vi "TurnXDegrees.vi"(8 "error in (no error)":errorcluster, 9 "Reset?":bool, 10 "degrees":dbl, 11 "RobotDriveDevRef":T1={"DevStatus"={"status"=FALSE, "code"=0, "source"=""}, "Motors[]"=[], "Square Inputs"=FALSE, "Max Output"=1.0, "Isochronous"=FALSE}) -> (0 "error out":errorcluster, 2 "Running":bool)   [LabVIEW 2013]
uses:
  <vilib>/Rock Robotics/WPI/RobotDrive/WPI_RobotDriveDevRef.ctl
  <vilib>/Rock Robotics/WPI/MotorControl/WPI_MotorControlDeviceRef.ctl
  <vilib>/Rock Robotics/SystemInterfaces/Typedef/FPGA_TypedefDigitalModule.ctl
  <vilib>/Rock Robotics/SystemInterfaces/DIO/FPGA_DIOPWMChannel.ctl
  <vilib>/Rock Robotics/WPI/PWM/WPI_PWMDeadband.ctl
  <vilib>/Rock Robotics/WPI/CAN/Jaguar/SubVIs/WPI_CANJaguar_ControlMode.ctl
  <vilib>/Rock Robotics/WPI/PWM/WPI_PWMTransform_ConPane.ctl
  <vilib>/addons/control/pid/pid.llb/PID Control Input Filter (DBL).vi
  <vilib>/addons/control/pid/pid.llb/PID (DBL).vi
  <vilib>/Rock Robotics/WPI/RobotDrive/WPI_RobotDriveArcadeDrive_Standard(NoSaturation).vi
  <vilib>/addons/control/pid/NI_PID_pid.lvlib
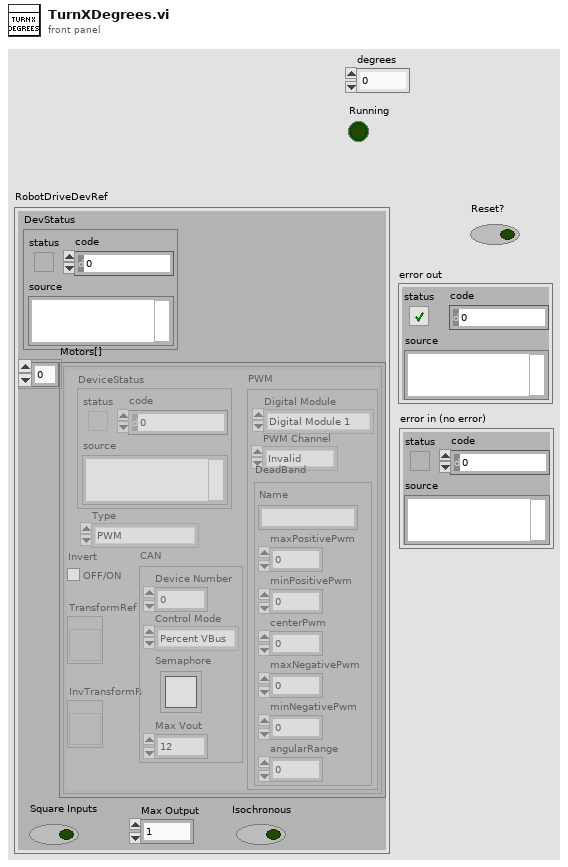
[diagram p1: front panel]
types:
  T1 = typedef "WPI_RobotDriveDevRef.ctl" = cluster{"DevStatus":errorcluster, "Motors[]":T2[], "Square Inputs":bool, "Max Output":dbl, "Isochronous":bool}
  T2 = typedef "WPI_MotorControlDeviceRef.ctl" = cluster{"DeviceStatus":errorcluster, "Type":enum16{"PWM", "CAN"}, "PWM":cluster{"Digital Module":T3, "PWM Channel":T4, "DeadBand":T5}, "CAN":cluster{"Device Number":u8, "Control Mode":T6, "Semaphore":T7, "Max Vout":dbl}, "Invert":bool, "TransformRef":T8, "InvTransformRef":T8}
  T3 = typedef "FPGA_TypedefDigitalModule.ctl" = enum16{"Digital Module 1", "Digital Module 2"}
  T4 = typedef "FPGA_DIOPWMChannel.ctl" = enum8{"PWM 1", "PWM 2", "PWM 3", "PWM 4", "PWM 5", "PWM 6", "PWM 7", "PWM 8", "PWM 9", "PWM 10", "Invalid"}
  T5 = typedef "WPI_PWMDeadband.ctl" = cluster{"Name":string, "maxPositivePwm":i32, "minPositivePwm":i32, "centerPwm":i32, "maxNegativePwm":i32, "minNegativePwm":i32, "angularRange":u16}
  T6 = typedef "WPI_CANJaguar_ControlMode.ctl" = enum8{"Percent VBus", "Current", "Speed", "Position", "Voltage"}
  T7 = typedef "Semaphore RefNum" = refnum<k1>
  T8 = typedef "WPI_PWMTransform_ConPane.ctl" = refnum<vi>
  T9 = cluster{"proportional gain (Kc)":dbl, "integral time (Ti, min)":dbl, "derivative time (Td, min)":dbl}
  T10 = typedef "WPI_GyroDevRef.ctl" = cluster{"DevStatus":errorcluster, "Analog Module":T11, "Analog Channel":T12, "Offset":dbl, "Gain (VoltsPerDegree/Second)":dbl}
  T11 = typedef "FPGA_TypedefAnalogModule.ctl" = enum16{"Analog Module 1", "Analog Module 2"}
  T12 = typedef "FPGA_AIChannel.ctl" = enum8{"AI 1", "AI 2", "AI 3", "AI 4", "AI 5", "AI 6", "AI 7", "AI 8", "Invalid"}
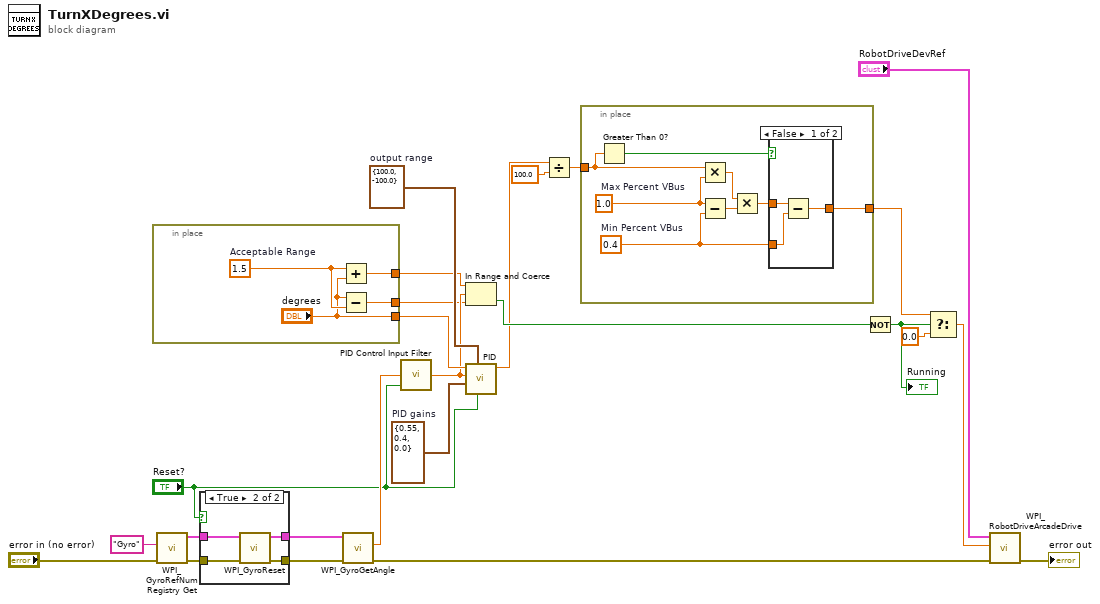
[diagram p0: block diagram]
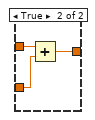
[diagram p2: hidden frame]
diagram:
  w15 = T9 {"proportional gain (Kc)"=0.55, "integral time (Ti, min)"=0.4, "derivative time (Td, min)"=0.0}  # PID gains
  w16 = cluster{"output high":dbl, "output low":dbl} {"output high"=100.0, "output low"=-100.0}  # output range
  n1 = in-place {
    in-place-border: [w28] -> w10
    in-place-border: [w27] -> w9
    in-place-border: ["degrees"] -> w12
    w29 = 1.5  # Acceptable Range
    n2 = Add(x=w29, y="degrees") -> (x+y=w28:dbl)
    n3 = Subtract(x="degrees", y=w29) -> (x-y=w27:dbl)
  }
  n4 = call <vilib>:"WPI_GyroRefNum Registry Get.vi"("error in (no error)"="error in (no error)", "refnum name"="Gyro") -> ("error out"=w21:errorcluster, "GyroDevRef"=w22:T10)  [unwired: 8 in]
  n5 = case shown="True" "Reset?" {
    tunnel: w22 -> [w31 w34]
    tunnel: w21 -> [w30 w35]
    tunnel: [w31 w33] -> w19
    tunnel: [w30 w32] -> w20
    frame False {
    }
    frame True {
      n6 = call <vilib>:"WPI_GyroReset.vi"("error in (no error)"=w35, "GyroDevRef"=w34) -> ("error out"=w32:errorcluster, "GyroDevRef"=w33:T10)  [unwired: 8 in]
    }
  }
  n7 = call <vilib>:"WPI_GyroGetAngle.vi"("error in (no error)"=w20, "GyroDevRef"=w19) -> ("error out"=w14:errorcluster, "Angle"=w18:dbl)  [unwired: 6 in, 2 out]
  n8 = call-poly <vilib>:"PID Control Input Filter.vi"("reinitialize? (F)"="Reset?", "input"=w18) -> ("output"=w11:dbl)  [unwired: 3 in]
  n9 = In Range and Coerce(upper limit=w10, x=w11, lower limit=w9) -> (In Range?=w8:bool)  [unwired: 1 out]
  n10 = call-poly <vilib>:"PID.vi"("reinitialize? (F)"="Reset?", "output range"=w16, "PID gains"=w15, "process variable"=w11, "setpoint"=w12) -> ("output"=w7:dbl)  [unwired: 5 in, 1 out]
  n11 = Divide(x=w7, y=100.0) -> (x/y=w6:dbl)
  n12 = in-place {
    in-place-border: [w41] -> w1
    in-place-border: w6 -> [w37]
    w39 = 0.4  # Min Percent VBus
    w38 = 1.0  # Max Percent VBus
    n13 = Greater Than 0?(x=w37) -> (x > 0?=w36:bool)
    n14 = Multiply(x=w37, y=w38) -> (x*y=w43:dbl)
    n15 = Subtract(x=w38, y=w39) -> (x-y=w40:dbl)
    n16 = Multiply(x=w43, y=w40) -> (x*y=w42:dbl)
    n17 = case shown="False" w36 {
      tunnel: w42 -> [w46 w49]
      tunnel: [w44 w48] -> w41
      tunnel: w39 -> [w45 w47]
      frame False {
        n18 = Subtract(x=w46, y=w45) -> (x-y=w44:dbl)
      }
      frame True {
        n19 = Add(x=w49, y=w47) -> (x+y=w48:dbl)
      }
    }
  }
  n20 = Not(x=w8) -> (.not. x?=w3:bool)
  "Running" <- w3
  n21 = Select(t=w1, s=w3, f=0.0 ("t")) -> (s? t:f=w4:dbl)
  n22 = call-poly <vilib>:"WPI_RobotDriveArcadeDrive.vi"("error in (no error)"=w14, "X axis value"=w4, "RobotDriveDevRef"="RobotDriveDevRef") -> ("error out"=→"error out":errorcluster)  [unwired: 6 in, 2 out]
